vi "init_instruments.vi"(8 "error in (no error)":errorcluster, 11 "UI_in":T1) -> (0 "error out":errorcluster, 3 "UI_out":T1)   [LabVIEW 2017]
uses:
  ui.ctl
  classes/dc_power_supply/DC_power_supply.lvclass
  classes/report/Report.lvclass
  ui_buttons.ctl
  types/boc_type.ctl
  <instrlib>/Siglent SDG X Series/Siglent SDG X Series.lvlib
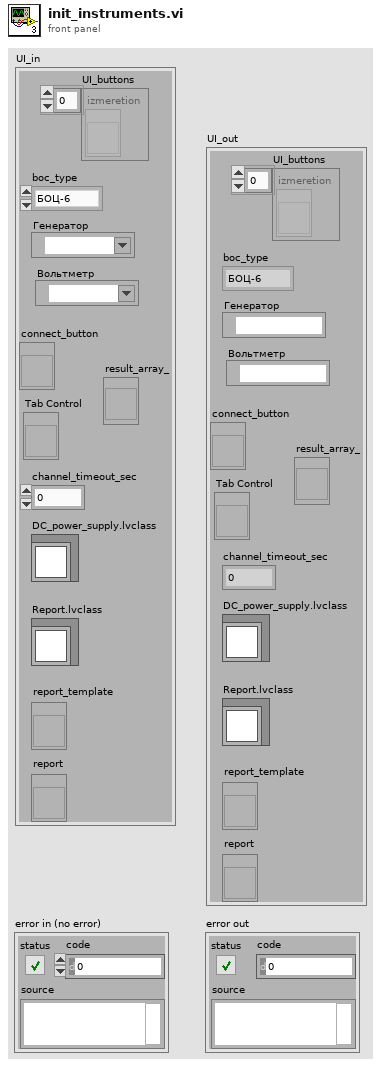
[diagram p1: front panel]
types:
  T1 = typedef "ui.ctl" = cluster{"UI_buttons":T2, "Tab Control":refnum<vi>, "connect_button":refnum<vi>, "generator":refnum<visa-resource-name>, "voltmetr":refnum<visa-resource-name>, "channel_timeout_sec":dbl, "boc_type":T3, "result_array_":refnum<vi>, "DC_power_supply.lvclass":refnum<class "DC_power_supply.lvclass">, "Report.lvclass":refnum<class "Report.lvclass">, "report_template":refnum<vi>, "report":refnum<vi>}
  T2 = typedef "ui_buttons.ctl" = refnum<vi>[]
  T3 = typedef "boc_type.ctl" = enum16{"БОЦ-6", "БОЦ-12"}
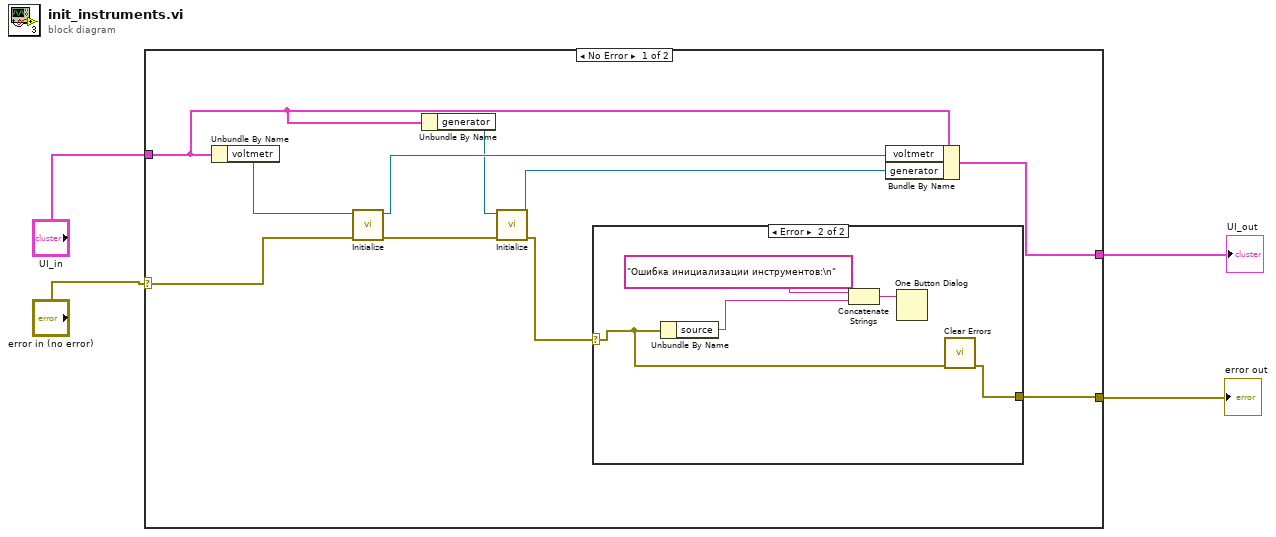
[diagram p0: block diagram]
diagram:
  n1 = case shown="No Error" "error in (no error)" {
    selector: "error in (no error)" -> [w7 w22]
    tunnel: [w14 w21] -> w4
    tunnel: [w6 w22] -> w3
    tunnel: "UI_in" -> [w9 w21]
    frame No Error {
      n2 = Unbundle By Name(w9) -> ("voltmetr"=w12:refnum<visa-resource-name>)
      n3 = call <instrlib>:"Initialize.vi"("error in (no error)"=w7, "VISA resource name"=w12) -> ("error out"=w11:errorcluster, "VISA resource name out"=w10:refnum<visa-resource-name>)  [unwired: 7 in, 1 out]
      n4 = Unbundle By Name(w9) -> ("generator"=w8:refnum<visa-resource-name>)
      n5 = call <instrlib>:"Initialize.vi"("error in (no error)"=w11, "VISA resource name"=w8) -> ("error out"=w5:errorcluster, "VISA resource name out"=w13:refnum<visa-resource-name>)  [unwired: 8 in]
      n6 = case shown="Error" w5 {
        selector: w5 -> [w15 w17]
        tunnel: [w15 w16] -> w6
        frame No Error {
        }
        frame Error {
          n7 = Unbundle By Name(w17) -> ("source"=w18:string)
          n8 = Concatenate Strings("Ошибка инициализации инструментов:\n" ("string"), w18) -> (w20:string)
          n9 = One Button Dialog(message=w20) -> ()  [unwired: 1 in, 1 out]
          n10 = call <vilib>:"Clear Errors.vi"("error in (no error)"=w17) -> ("error out"=w16:errorcluster)  [unwired: 5 in, 1 out]
        }
      }
      n11 = Bundle By Name(cluster=w9, "voltmetr"=w10, "generator"=w13) -> (w14:T1)
    }
    frame Error {
    }
  }
  "UI_out" <- w4
  "error out" <- w3
